vi "Set motor RPM.vi"(3 "RPM (/min)":dbl, 4 "Drive address":T3=1 items=["0", "1", "2", "3", "4", "5", "6", "7", "8", "9", "10", "11", "12", "13", "14", "15", "16", "17", "18", "19", "20", "21", "22", "23", "24", "25", "26", "27", "28", "29", "30", "31", "32", "33", "34", "35", "36", "37", "38", "39", "40", "41", "42", "43", "44", "45", "46", "47", "48", "49", "50", "51", "52", "53", "54", "55", "56", "57", "58", "59", "60", "61", "62", "63"], 5 "COM port":refnum<visa-resource-name>) -> (1 "Modbus error cluster":T1={"Checksum ok"=FALSE, "Modbus exception code"=1, "Response from correct drive"=FALSE, "Comms error"={"status"=FALSE, "code"=0, "source"=""}} {"Modbus exception code" items=["None"=0, "Invalid function request"=1, "Invalid Modbus register address"=2, "Invalid / unauthorised data value"=3, "Device failure"=4, "Request accepted, wait"=5, "Drive busy"=6, "Request rejected"=7, "Memory parity error"=8, "Gateway path unavailable"=10, "Device failed to respond"=11]}, 2 "No errors":bool)   [LabVIEW 2020]
doc: "Modbus RTU for Invertek drives. Paul Nathan 21-JUN-2022."
uses:
  ctls/Drive address.ctl
  ctls/Register.ctl
  Globals/Invertek Drive Params.vi
  ctls/Exception codes.ctl
  ctls/Modbus error cluster.ctl
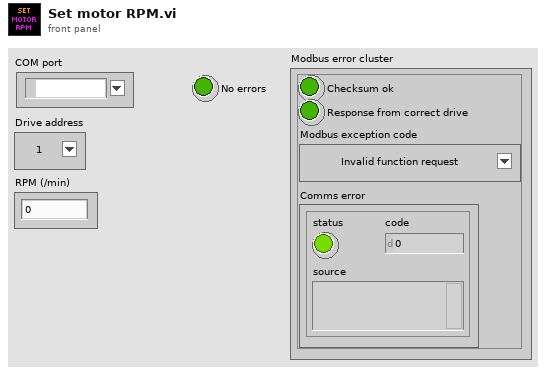
[diagram p1: front panel]
types:
  T1 = typedef "Modbus error cluster.ctl" = cluster{"Checksum ok":bool, "Modbus exception code":T2, "Response from correct drive":bool, "Comms error":errorcluster}
  T2 = typedef "Exception codes.ctl" = u8
  T3 = typedef "Drive address.ctl" = u8
  T4 = typedef "Register.ctl" = u16
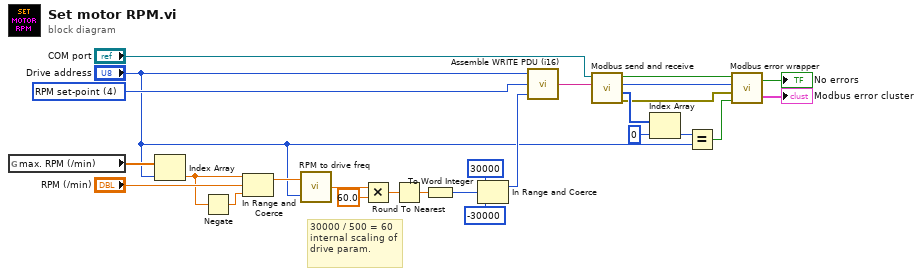
[diagram p0: block diagram]
diagram:
  w15 = T4 4 items=["Control"=0, "RPM set-point"=4, "Drive status"=5, "Output RPM"=6, "Motor current"=7, "Motor torque"=8, "Motor power"=9, "DC bus voltage"=22, "Drive power stage temperature"=23, "kWh meter"=31, "MWh meter"=32, "Running time - hours"=33, "Running time - seconds"=34, "Internal drive temperature"=38, "Motor RMS voltage"=42, "Extended drive status"=2000] ("Register")
  # "30000 / 500 = 60 internal scaling of drive param."
  n1 = global read "Invertek Drive Params.vi" "max. RPM (/min)"() -> (w9:dbl[])
  n2 = Index Array(array=w9, index="Drive address") -> (element=w8:dbl)
  n3 = Negate(x=w8) -> (-x=w10:dbl)
  n4 = In Range and Coerce(upper limit=w8, x="RPM (/min)", lower limit=w10) -> (coerced(x)=w11:dbl)  [unwired: 1 out]
  n5 = call "RPM to drive freq.vi"("Drive address"="Drive address", "Motor RPM (/min)"=w11) -> ("Drive output f (Hz)"=w14:dbl)
  n6 = Multiply(x=w14, y=60.0) -> (x*y=w21:dbl)
  n7 = Round To Nearest(number=w21) -> (nearest integer value=w20:dbl)
  n8 = To Word Integer(number=w20) -> (16bit integer=w19:i16)
  n9 = In Range and Coerce(upper limit=i16 30000, x=w19, lower limit=i16 -30000) -> (coerced(x)=w18:i16)  [unwired: 1 out]
  n10 = call "Assemble WRITE PDU (i16).vi"("i16 value"=w18, "Register"=w15, "Drive address"="Drive address") -> ("Ser out string"=w26:string)
  n11 = call "Modbus send and receive.vi"("Modbus telegram"=w26, "COM port"="COM port") -> ("Comms error"=w2:errorcluster, "Device response"=w24:u8[], "Modbus exception code"=w1:T2, "Checksum ok"=w4:bool)  [unwired: 2 in]
  n12 = Index Array(array=w24, index=0) -> (element=w22:u8)
  n13 = Equal?(x=w22, y="Drive address") -> (x = y?=w3:bool)
  n14 = call "Modbus error wrapper.vi"("Response from correct drive"=w3, "Comms error"=w2, "Modbus exception code"=w1, "Checksum ok"=w4) -> ("Modbus error cluster"=→"Modbus error cluster":T1, "No errors"=→"No errors":bool)
